vi "plot_graph.vi"() -> ()   [LabVIEW 2020]
panel:
  out "XY Graph 2":cluster{dbl[], dbl[]}(graph)
  out "Numeric":i32
  out "XY Graph":cluster{dbl[], dbl[]}[](graph)
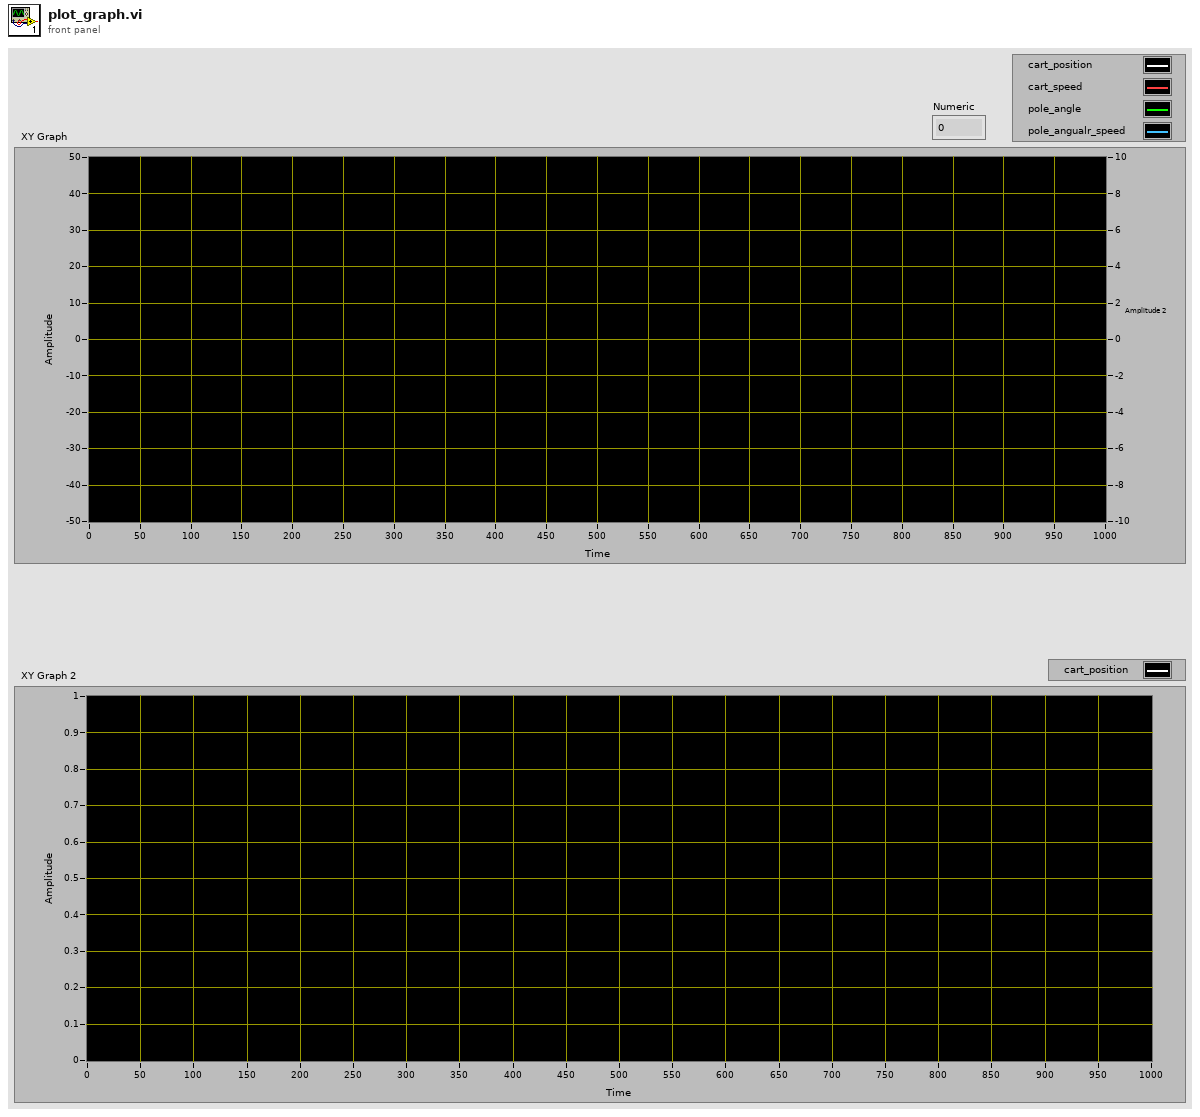
[diagram p1: front panel]
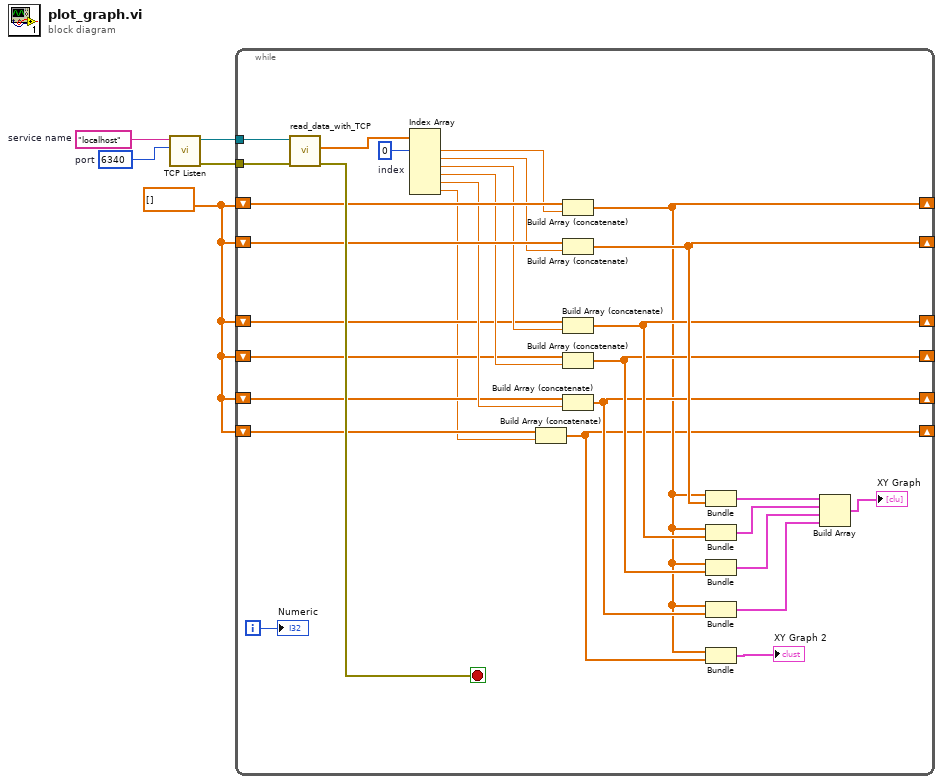
[diagram p0: block diagram]
diagram:
  w1 = dbl[] []
  w4 = u16 6340  # port
  w5 = "localhost"  # service name
  n1 = call <vilib>:"TCP Listen.vi"("port"=w4, "service name"=w5) -> ("error out"=w2:errorcluster, "connection ID"=w3:refnum<k5>)  [unwired: 5 in, 3 out]
  n2 = while {
    tunnel: w3 -> [w35]
    tunnel: w2 -> [w34]
    shift-right: [w8] -> _
    shift-left: w1 -> [w30]
    shift-right: [w28] -> _
    shift-left: w1 -> [w29]
    shift-right: [w14] -> _
    shift-left: w1 -> [w17]
    shift-right: [w13] -> _
    shift-left: w1 -> [w16]
    shift-right: [w12] -> _
    shift-left: w1 -> [w15]
    shift-right: [w7] -> _
    shift-left: w1 -> [w10]
    i -> [w11]
    stop <- w33 stop-if-true
    w31 = 0  # index
    n3 = call "read_data_with_TCP.vi"("error_in"=w34, "TCP_ref_in"=w35) -> ("error_out"=w33:errorcluster, "data_out"=w32:dbl[])  [unwired: 7 in, 1 out]
    n4 = Index Array(array=w32, index #1=w31) -> (element #1=w27:dbl, element #2=w26:dbl, element #3=w20:dbl, element #4=w19:dbl, element #5=w18:dbl, element #6=w9:dbl)  [unwired: 5 in]
    n5 = Build Array (concatenate)(w10, w9) -> (w7:dbl[])
    n6 = Build Array (concatenate)(w30, w27) -> (w8:dbl[])
    n7 = Build Array (concatenate)(w29, w26) -> (w28:dbl[])
    n8 = Build Array (concatenate)(w17, w20) -> (w14:dbl[])
    n9 = Build Array (concatenate)(w16, w19) -> (w13:dbl[])
    n10 = Build Array (concatenate)(w15, w18) -> (w12:dbl[])
    n11 = Bundle(w8, w28) -> (w25:cluster{dbl[], dbl[]})  [unwired: 1 in]
    n12 = Bundle(w8, w14) -> (w23:cluster{dbl[], dbl[]})  [unwired: 1 in]
    n13 = Bundle(w8, w13) -> (w22:cluster{dbl[], dbl[]})  [unwired: 1 in]
    n14 = Bundle(w8, w12) -> (w21:cluster{dbl[], dbl[]})  [unwired: 1 in]
    n15 = Bundle(w8, w7) -> (→"XY Graph 2":cluster{dbl[], dbl[]})  [unwired: 1 in]
    n16 = Build Array(w25, w23, w22, w21) -> (→"XY Graph":cluster{dbl[], dbl[]}[])
    "Numeric" <- w11
  }
